vi "Read Encoding.vi"(11 "ConfigManager in":refnum<class "ConfigManager.lvclass">) -> (2 "Encoding":refnum<class "Encoding.lvclass">, 3 "ConfigManager out":refnum<class "ConfigManager.lvclass">)   [LabVIEW 2013, in "SMOConfig.lvlib" / "ConfigManager.lvclass"]
uses:
  ConfigManager.lvclass
  Encoding/Encoding.lvclass
  ConfigManager.lvclass/ConfigManager.ctl
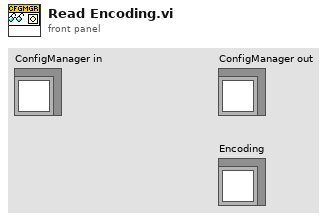
[diagram p1: front panel]
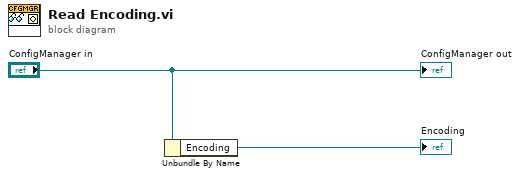
[diagram p0: block diagram]
diagram:
  n1 = Unbundle By Name("ConfigManager in") -> ("Encoding"=→"Encoding":refnum<class "Encoding.lvclass">)
  "ConfigManager out" <- "ConfigManager in"
